vi "PV reconnect status checking.vi"() -> (2 "failure_flag 4":bool)   [LabVIEW 2016]
uses:
  Communication/Global communication.vi
panel:
  out "Boolean 2":bool
  in  "i>=20?":bool
  in  "=1?":bool
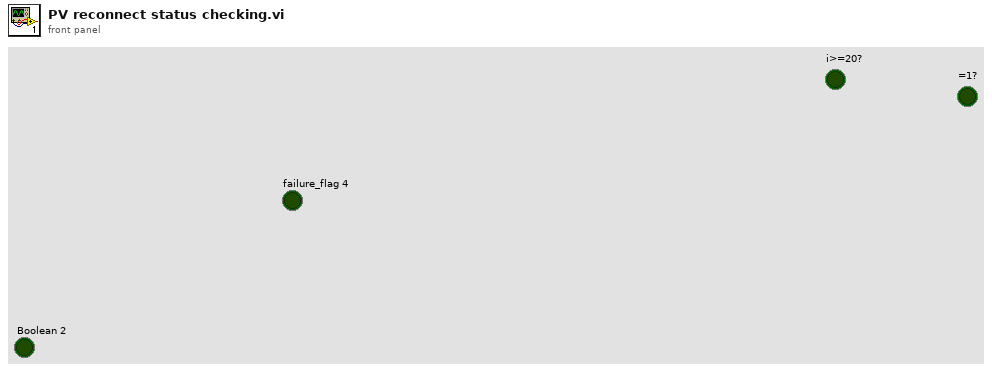
[diagram p1: front panel]
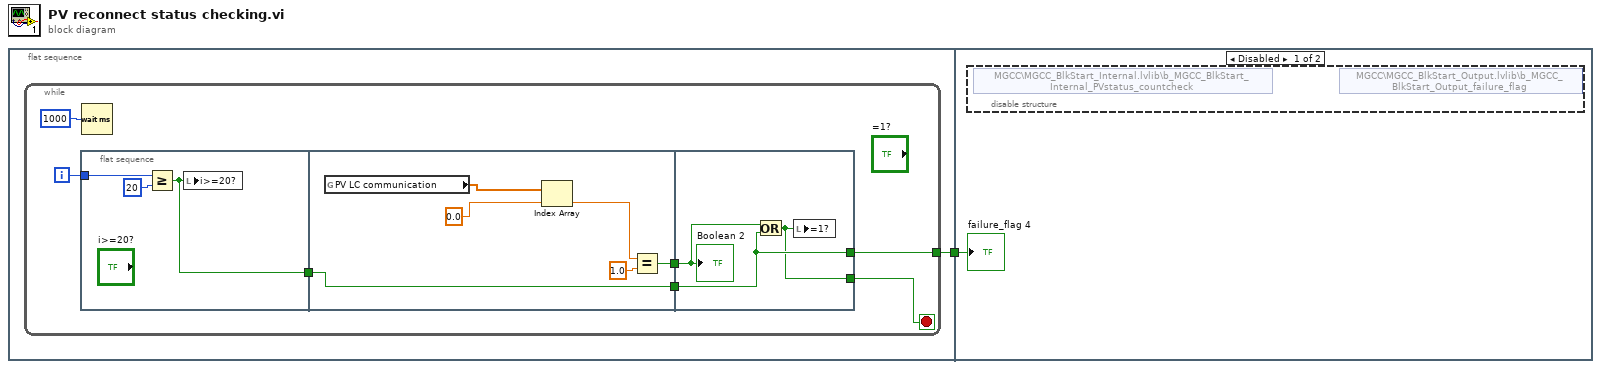
[diagram p0: block diagram]
diagram:
  n1 = flat-sequence {
    tunnel: [w2] -> w1
    tunnel: w1 -> [w22]
    frame #0 {
      n2 = while {
        tunnel: [w5] -> w2
        i -> [w8]
        stop <- w3 stop-if-true
        n3 = flat-sequence {
          tunnel: w8 -> [w12]
          tunnel: [w10] -> w4
          tunnel: [w18] -> w7
          tunnel: [w16] -> w6
          tunnel: w4 -> [w18]
          tunnel: w7 -> [w20]
          tunnel: w6 -> [w21]
          tunnel: [w20] -> w5
          tunnel: [w19] -> w3
          frame #0 {
            n4 = Greater Or Equal?(x=w12, y=20) -> (x >= y?=w10:bool)
            n5 = local write "i>=20?"(w10) -> ()
          }
          frame #1 {
            n6 = global read "Global communication.vi" "PV LC communication"() -> (w13:dbl[])
            n7 = Index Array(array=w13, index=0.0) -> (element=w14:dbl)
            n8 = Equal?(x=w14, y=1.0) -> (x = y?=w16:bool)
          }
          frame #2 {
            n9 = Or(x=w21, y=w20) -> (x .or. y?=w19:bool)
            n10 = local write "=1?"(w19) -> ()
            "Boolean 2" <- w21
          }
        }
        n11 = Wait (ms)(milliseconds to wait=1000) -> ()  [unwired: 1 out]
      }
    }
    frame #1 {
      n12 = disable-structure shown="Disabled" {
        frame Disabled {
          n13 = shared-variable "MGCC\\MGCC_BlkStart_Internal.lvlib\\b_MGCC_BlkStart_Internal_PVstatus_countcheck"() -> ()  [unwired: 1 in, 2 out]
          n14 = shared-variable "MGCC\\MGCC_BlkStart_Output.lvlib\\b_MGCC_BlkStart_Output_failure_flag"() -> ()  [unwired: 2 in, 1 out]
        }
        frame Enabled {
        }
      }
      "failure_flag 4" <- w22
    }
  }
